vi "createILCDAC.vi"(8 "error in (no error)":errorcluster, 10 "Channel":u8=1 min=1 max=4, 11 "ILCDACFactory in":refnum<class "ILCDACFactory.lvclass">) -> (0 "error out":errorcluster, 2 "ILCDAC":refnum<class "IILCDAC.lvclass">, 3 "ILCDACFactory out":refnum<class "ILCDACFactory.lvclass">)   [LabVIEW 2015, in "ILCDACFactory.lvclass"]
uses:
  ILCDACFactory.lvclass
  ILCDAC/ILCDAC1/ILCDAC1.lvclass
  ILCDAC/ILCDAC2/ILCDAC2.lvclass
  ILCDAC/ILCDAC3/ILCDAC3.lvclass
  ILCDAC/ILCDAC4/ILCDAC4.lvclass
  ILCDAC/IILCDAC/IILCDAC.lvclass
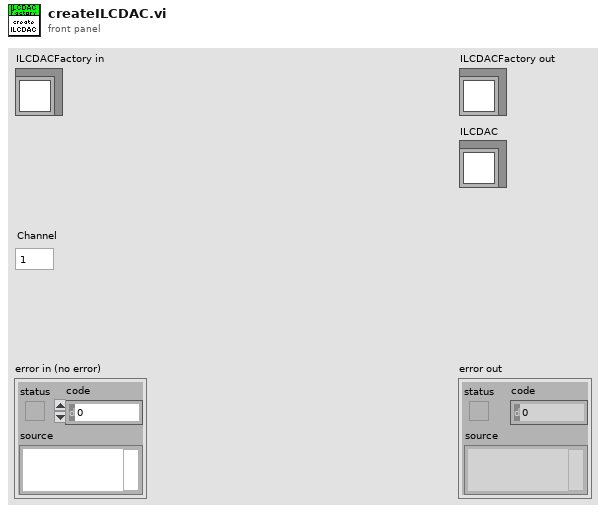
[diagram p1: front panel]
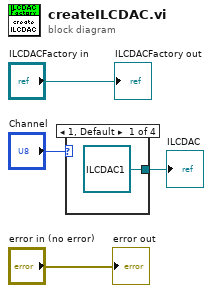
[diagram p0: block diagram]
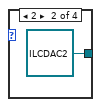
[diagram p2: hidden frame]
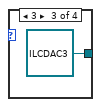
[diagram p3: hidden frame]
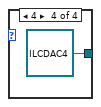
[diagram p4: hidden frame]
diagram:
  n1 = case shown="1, Default" "Channel" {
    tunnel: [refnum<class "ILCDAC1.lvclass"> refnum ("ILCDAC1.lvclass") refnum<class "ILCDAC2.lvclass"> refnum ("ILCDAC2.lvclass") refnum<class "ILCDAC3.lvclass"> refnum ("ILCDAC3.lvclass") refnum<class "ILCDAC4.lvclass"> refnum ("ILCDAC4.lvclass")] -> w1
    frame 1, Default {
    }
    frame 2 {
    }
    frame 3 {
    }
    frame 4 {
    }
  }
  "ILCDAC" <- w1
  "error out" <- "error in (no error)"
  "ILCDACFactory out" <- "ILCDACFactory in"
